vi "queue.vi"(7 "action":string="Enqueue", 8 "error_in":errorcluster, 11 "element_in":string) -> (0 "error_out":errorcluster, 3 "element_out":string)   [LabVIEW 2018]
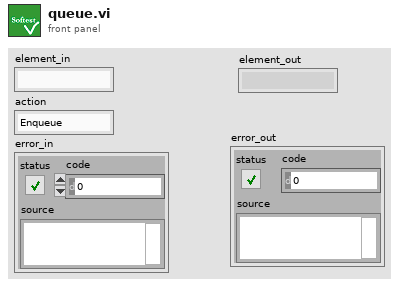
[diagram p1: front panel]
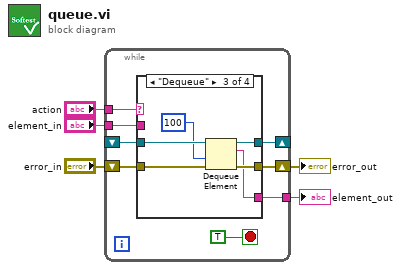
[diagram p0: block diagram]
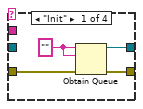
[diagram p2: hidden frame]
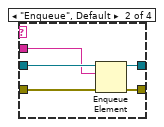
[diagram p3: hidden frame]
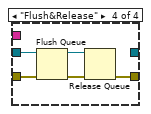
[diagram p4: hidden frame]
diagram:
  n1 = while {
    shift-right: [w12] -> w2
    shift-left: "error_in" -> [w11]
    tunnel: "action" -> [w10]
    shift-right: [w9] -> _
    shift-left: _ -> [w8]
    tunnel: "element_in" -> [w7]
    tunnel: [w6] -> w3
    stop <- TRUE stop-if-true
    n2 = case shown="\"Dequeue\"" w10 {
      tunnel: [w17 w22 w27 w33] -> w12
      tunnel: w11 -> [w15 w21 w28 w32]
      tunnel: [w16 w20 w26 _] -> w9
      tunnel: w8 -> [_ w19 w25 w30]
      tunnel: w7 -> [_ w18 _ _]
      tunnel: [_ _ w23 _] -> w6
      frame "Init" {
        w14 = ""
        n3 = Obtain Queue(name (unnamed)=w14, element data type=w14, error in (no error)=w15) -> (queue out=w16:refnum<queue>, error out=w17:errorcluster)  [unwired: 2 in, 1 out]
      }
      frame "Enqueue", Default {
        n4 = Enqueue Element(queue=w19, element=w18, error in (no error)=w21) -> (queue out=w20:refnum<queue>, error out=w22:errorcluster)  [unwired: 1 in, 1 out]
      }
      frame "Dequeue" {
        n5 = Dequeue Element(queue=w25, timeout in ms (-1)=100, error in (no error)=w28) -> (queue out=w26:refnum<queue>, element=w23:string, error out=w27:errorcluster)  [unwired: 1 out]
      }
      frame "Flush&Release" {
        n6 = Flush Queue(queue=w30, error in (no error)=w32) -> (queue out=w29:refnum<queue>, error out=w31:errorcluster)  [unwired: 1 out]
        n7 = Release Queue(queue=w29, error in (no error)=w31) -> (error out=w33:errorcluster)  [unwired: 1 in, 2 out]
      }
    }
  }
  "element_out" <- w3
  "error_out" <- w2
